vi "Write Descr.vi"(8 "error in (no error)":errorcluster, 10 "Descr":T1, 11 "CRDS Cell in":refnum<class "CRDS Cell.lvclass">=refnum) -> (0 "error out":errorcluster, 3 "CRDS Cell out":refnum<class "CRDS Cell.lvclass">)   [LabVIEW 2012]
uses:
  CRDS Cell.lvclass
  PAS_CRDS new/CRDS/Controls/chDescr.ctl
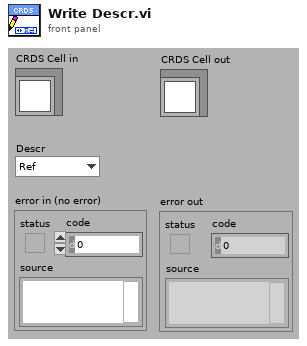
[diagram p1: front panel]
types:
  T1 = typedef "chDescr.ctl" = enum16{"Ref", "Dry", "60%", "90%"}
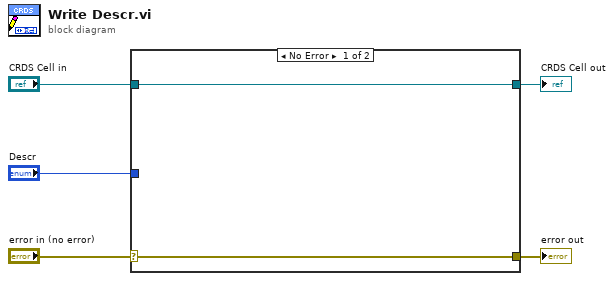
[diagram p0: block diagram]
diagram:
  n1 = case shown="No Error" "error in (no error)" {
    selector: "error in (no error)" -> [w7 w8]
    tunnel: [w7 w8] -> w4
    tunnel: [w6 w9] -> w2
    tunnel: "CRDS Cell in" -> [w6 w9]
    tunnel: "Descr" -> [_ _]
    frame No Error {
    }
    frame Error {
    }
  }
  "error out" <- w4
  "CRDS Cell out" <- w2
